vi "LVClass_SlopesPostProcessList Read SlopesPostProccessor.vi"(8 "error in (no error)":errorcluster, 11 "SlopesPostProcessorList in":refnum<class "SlopesPostProcessorList.lvclass">) -> (0 "error out":errorcluster, 2 "SlopesPostProccessor":i32, 3 "SlopesPostProcessorList out":refnum<class "SlopesPostProcessorList.lvclass">)   [LabVIEW 2020, in "SlopesPostProcessorList.lvclass"]
uses:
  SlopesPostProcessorList.lvclass
  SlopesPostProcessorList.lvclass/SlopesPostProcessorList.ctl
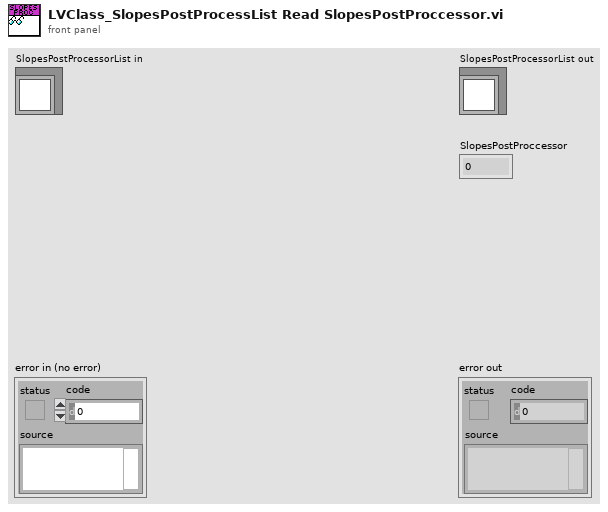
[diagram p1: front panel]
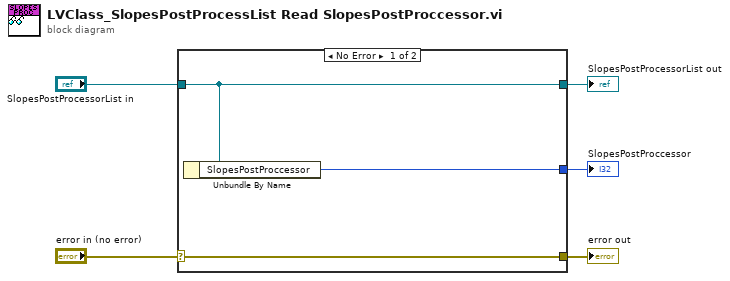
[diagram p0: block diagram]
diagram:
  n1 = case shown="No Error" "error in (no error)" {
    selector: "error in (no error)" -> [w8 w9]
    tunnel: [w8 w9] -> w4
    tunnel: [w7 w10] -> w2
    tunnel: "SlopesPostProcessorList in" -> [w7 w10]
    tunnel: [w6 _] -> w1
    frame No Error {
      n2 = Unbundle By Name(w7) -> ("SlopesPostProccessor"=w6:i32)
    }
    frame Error {
    }
  }
  "error out" <- w4
  "SlopesPostProcessorList out" <- w2
  "SlopesPostProccessor" <- w1
